vi "Envelope.vi"(0 "IN":dbl[](array[numeric]), 3 "Release":dbl, 4 "Decay":dbl, 5 "Sustain Level":dbl, 7 "Attack":dbl, 10 "SampleLenght":dbl) -> (20 "OUT":dbl[](array[numeric]))   [LabVIEW 2025]
uses:
  <vilib>/Analysis/NI_AALBase.lvlib
  <vilib>/Analysis/1siggen.llb/Ramp Pattern by Samples.vi
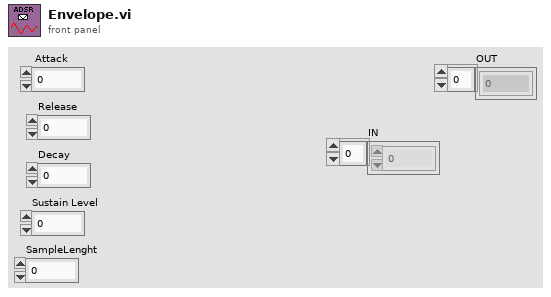
[diagram p1: front panel]
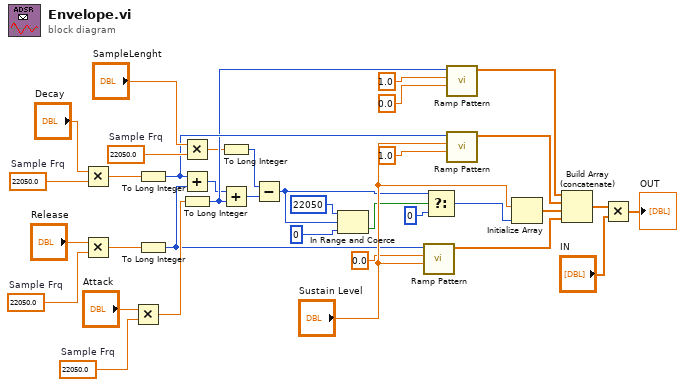
[diagram p0: block diagram]
diagram:
  w4 = 22050.0  # Sample Frq
  w3 = 22050.0  # Sample Frq
  w2 = 22050.0  # Sample Frq
  w35 = 22050.0  # Sample Frq
  n1 = Multiply(x="Decay", y=w4) -> (x*y=w26:dbl)
  n2 = Multiply(x="Release", y=w3) -> (x*y=w25:dbl)
  n3 = Multiply(x="Attack", y=w2) -> (x*y=w24:dbl)
  n4 = To Long Integer(number=w26) -> (32bit integer=w29:i32)
  n5 = To Long Integer(number=w25) -> (32bit integer=w17:i32)
  n6 = Multiply(x="SampleLenght", y=w35) -> (x*y=w7:dbl)
  n7 = Add(x=w29, y=w17) -> (x+y=w5:i32)
  n8 = To Long Integer(number=w24) -> (32bit integer=w28:i32)
  n9 = To Long Integer(number=w7) -> (32bit integer=w8:i32)
  n10 = Add(x=w5, y=w28) -> (x+y=w6:i32)
  n11 = Subtract(x=w8, y=w6) -> (x-y=w11:i32)
  n12 = In Range and Coerce(upper limit=22050, x=w11, lower limit=0) -> (In Range?=w10:bool)  [unwired: 1 out]
  n13 = call-poly <vilib>:"Ramp Pattern.vi"("start"="Sustain Level", "end"=0.0, "samples"=w17) -> ("Ramp Pattern"=w22:dbl[])  [unwired: 7 in, 1 out]
  n14 = Select(t=w11, s=w10, f=0) -> (s? t:f=w16:i32)
  n15 = call-poly <vilib>:"Ramp Pattern.vi"("start"=0.0, "end"=1.0, "samples"=w28) -> ("Ramp Pattern"=w19:dbl[])  [unwired: 7 in, 1 out]
  n16 = call-poly <vilib>:"Ramp Pattern.vi"("start"=1.0, "end"="Sustain Level", "samples"=w29) -> ("Ramp Pattern"=w20:dbl[])  [unwired: 7 in, 1 out]
  n17 = Initialize Array("Sustain Level", w16) -> (w21:dbl[])
  n18 = Build Array (concatenate)(w19, w20, w21, w22) -> (w23:dbl[])
  n19 = Multiply(x=w23, y="IN") -> (x*y=→"OUT":dbl[])
